vi "Read Single U16 Image and Metadata from file.vi"(7 "File":refnum<file>, 8 "error out":errorcluster, 9 "Tags":T2[](array[typedef]), 10 "Litt/BigEnd":bool, 11 "U16 Image":T1) -> (0 "error out":errorcluster, 3 "U16 Image (duplicate)":T1, 5 "File dup":refnum<file>)   [LabVIEW 2013, in "Tiff reader.lvlib"]
doc: "Read a single image and it's metadata from a file ref."
uses:
  Tiff reader.lvlib
  IFD Entry.ctl
  FieldTypes.ctl
  <vilib>/vision/Image Controls.llb/IMAQ Image.ctl
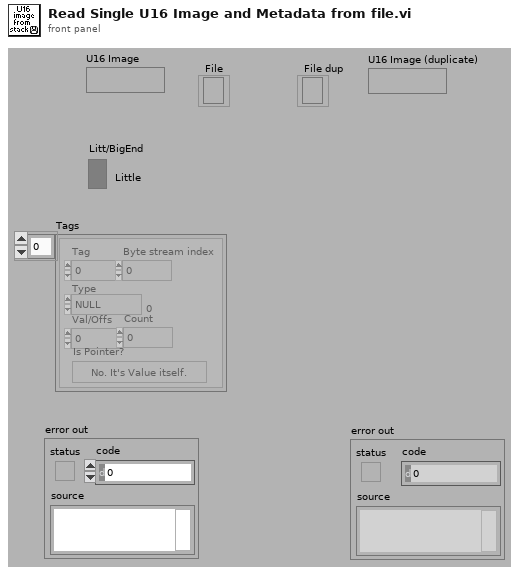
[diagram p1: front panel]
types:
  T1 = typedef "IMAQ Image.ctl" = refnum<image>
  T2 = typedef "Tiff reader.lvlib/IFD Entry.ctl" = cluster{"Tag":u16, "Type":T3, "Count":u32, "Val/Offs":u32, "Is Pointer?":bool, "Byte stream index":i32}
  T3 = typedef "Tiff reader.lvlib/FieldTypes.ctl" = enum16{"NULL", "U8", "ASCII7", "U16", "U32", "RATIONAL", "SByte(I8)", "Undef(8Bit)", "I16", "I32", "SRat(4B:4B)", "SGL(4Byte)", "DBL(8Byte)"}
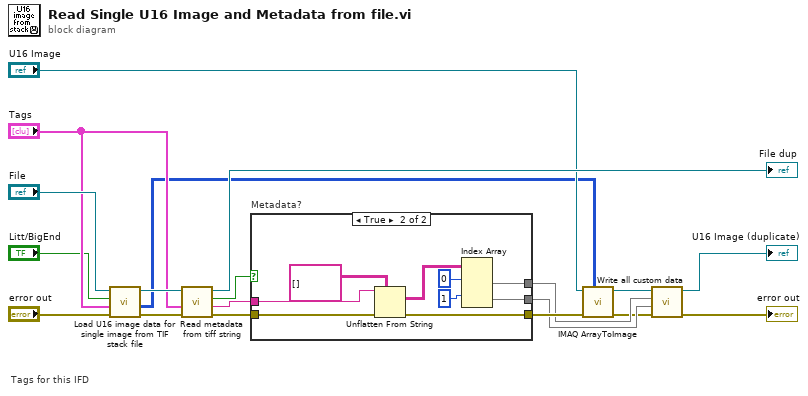
[diagram p0: block diagram]
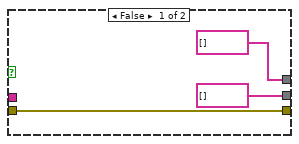
[diagram p2: hidden frame]
diagram:
  # "Tags for this IFD"
  n1 = call "Load U16 image data for single image from TIF stack file.vi"("error in"="error out", "DirEntries"="Tags", "Litt/BigEnd"="Litt/BigEnd", "File"="File") -> ("error out"=w3:errorcluster, "U16"=w1:u16[][], "File"=w7:refnum<file>)  [unwired: 5 in]
  n2 = call "Read metadata from tiff string.vi"("error in"=w3, "DirEntries"="Tags", "Tiff image stack"=w7) -> ("error out"=w16:errorcluster, "Metadata string"=w15:string, "Tag exists?"=w17:bool, "Tiff image stack dup"=→"File dup":refnum<file>)  [unwired: 1 in, 4 out]
  n3 = case "Metadata?" shown="True" w17 {
    tunnel: w15 -> [_ w31]
    tunnel: w16 -> [w22 w29]
    tunnel: [string[] [] w27] -> w12
    tunnel: [string[] [] w26] -> w14
    tunnel: [w22 w23] -> w19
    frame False {
    }
    frame True {
      n4 = Unflatten From String(type=string[][] [], binary string=w31, error in (no error)=w29) -> (value=w28:string[][], error out=w23:errorcluster)  [unwired: 3 out]
      n5 = Index Array(array=w28, index (row) #1=0 ("index (row)"), index (row) #2=1 ("index (row)")) -> (element #1=w27:string[], element #2=w26:string[])  [unwired: 2 in]
    }
  }
  n6 = call "IMAQ ArrayToImage"("Image Pixels (U16)"=w1, "error in (no error)"=w19, "Image"="U16 Image") -> ("error out"=w11:errorcluster, "Image Out"=w8:T1)  [unwired: 3 in, 4 out]
  n7 = call "Write all custom data.vi"("error in (no error)"=w11, "Custom Data"=w14, "Keys"=w12, "img"=w8) -> ("error out"=→"error out":errorcluster, "Image (duplicate)"=→"U16 Image (duplicate)":T1)  [unwired: 6 out]
